vi "PCM Panel With Menu UI.vi"() -> ()   [LabVIEW 2016, in "PCM PanelSplit.lvclass"]
uses:
  PCM PanelSplit.lvclass
  PanelSplitToolkit/PanelObject/PanelObject.lvclass
  SubClass/PCM MenuVIPanelSplit.lvclass
  C:/Users/CL/Desktop/ZcDAQprj0811/ZcDAQprj/Modules/DAQ-Display/PanelSplitToolkit/PanelRootNode/PanelRootNode.lvclass
  PanelSplitToolkit/PanelDataNode/Split Mode.ctl
  <vilib>/Utility/error.llb/DialogType.ctl
  Display Mode.ctl
  <vilib>/Analysis/4window.llb/windowTd.ctl
  PanelSplitToolkit/PanelDataNode/PanelDataNode.lvclass
  <vilib>/Utility/miscctls.llb/LVRangeTypeDef.ctl
  PanelSplitToolkit/QueueManager.llb/CreatQueue.vi
  PanelSplitToolkit/QueueManager.llb/Insert.vi
  PanelSplitToolkit/QueueManager.llb/Remove.vi
  PanelSplitToolkit/QueueManager.llb/Destroy.vi
  PanelSplitToolkit/PanelRootNode/PanelRootNode.lvclass
  <vilib>/Analysis/NI_AALPro.lvlib
panel:
  in  "History":bool
  in  "Setting":bool
  in  "Float":bool
  in  "Close":bool
  in  "Node*":refnum<data-value>
  in  "down":bool
  in  "right":bool
  in  "left":bool
  in  "up":bool
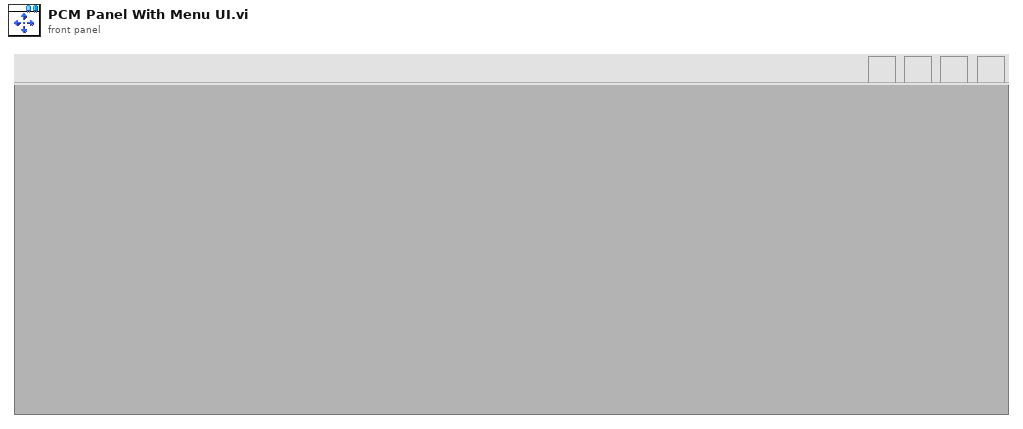
[diagram p1: front panel]
types:
  T1 = cluster{"Display[]":bool[], "error":errorcluster, "Float":bool}
  T2 = cluster{"error":errorcluster, "Event":string, "Data":variant, "Q_Local":string, "Caller":string, "SubPanel*":refnum<vi>, "RootNode*":refnum<data-value>, "Send":cluster{"SEvent":string, "SData":variant, "PanelNumber":i32}, "Arrow Button Refs":refnum<vi>[]}
  T3 = typedef "PanelDataNode.lvclass/Split Mode.ctl" = enum16{"Horizontal(up)", "Vertical(left)", "Horizontal(down)", "Vertical(right)"}
  T4 = typedef "LVPoint32TypeDef.ctl" = cluster{"Horizontal":i32, "Vertical":i32}
  T5 = typedef "PCM PanelSplit.lvclass/Display Mode.ctl" = enum16{"时域", "频谱", "功率谱"}
  T6 = enum32{"Invalid", "Standard", "Closed", "Hidden", "Minimized", "Maximized"}
  T7 = typedef "LVRangeTypeDef.ctl" = cluster{"Minimum":dbl, "Maximum":dbl, "Increment":dbl, "Minor Increment":dbl, "Start":dbl}
  T8 = typedef "DialogType.ctl" = u16
  T9 = typedef "PCM PanelSplit.lvclass/Display Config.ctl" = cluster{"Display Mode":T5, "ChTag[]":string[], "window":T10, "Range":T7}
  T10 = typedef "NI_AALPro.lvlib/windowTd.ctl" = u32
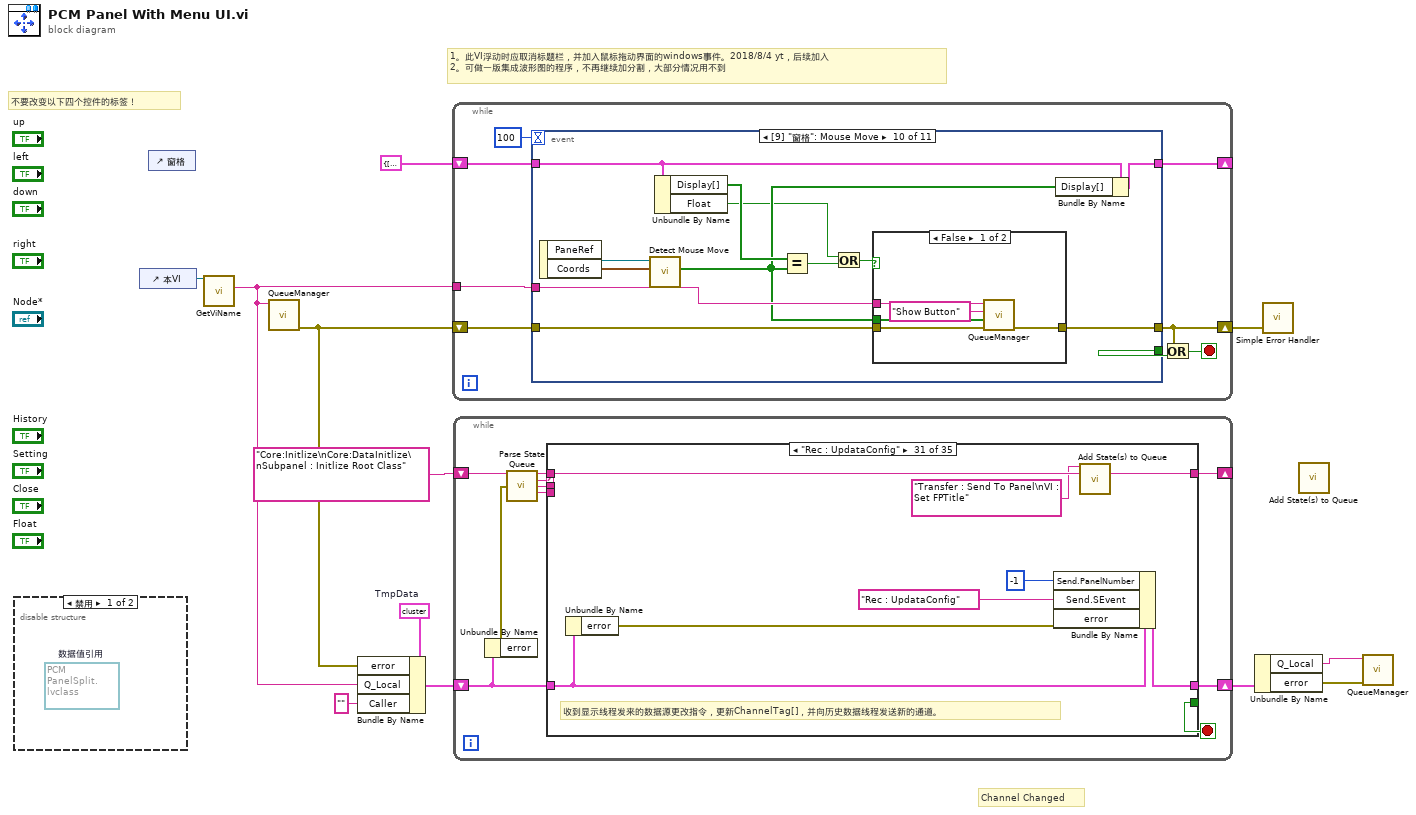
[diagram p0: block diagram]
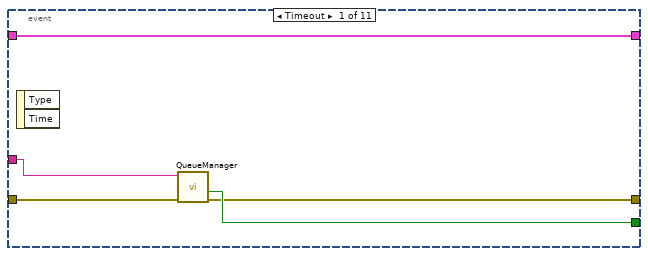
[diagram p3: hidden frame]
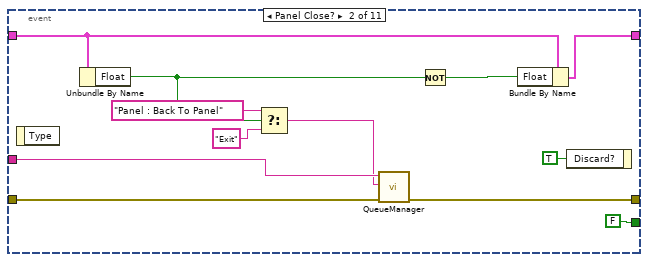
[diagram p4: hidden frame]
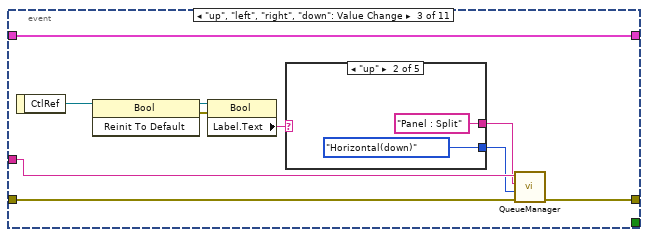
[diagram p5: hidden frame]
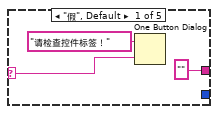
[diagram p6: hidden frame]
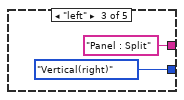
[diagram p7: hidden frame]
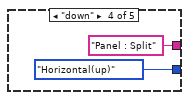
[diagram p8: hidden frame]
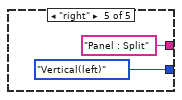
[diagram p9: hidden frame]
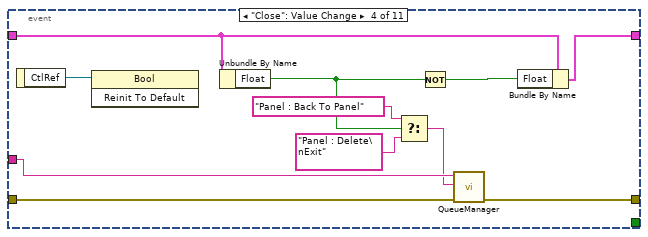
[diagram p10: hidden frame]
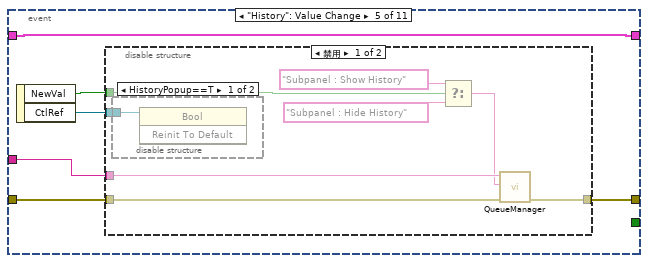
[diagram p11: hidden frame]
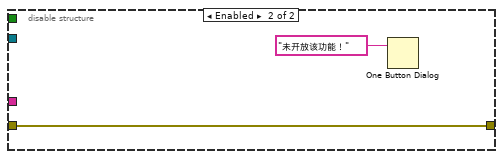
[diagram p13: hidden frame]
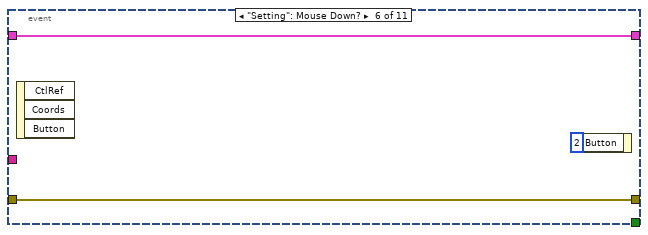
[diagram p14: hidden frame]
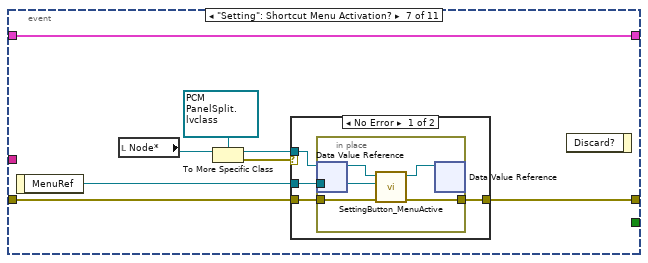
[diagram p15: hidden frame]
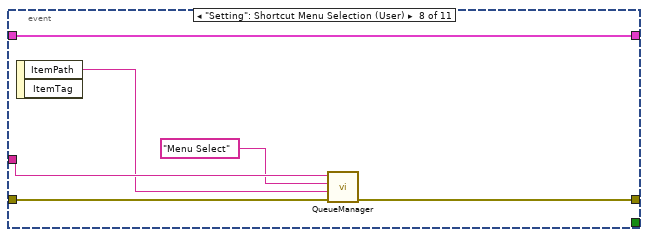
[diagram p17: hidden frame]
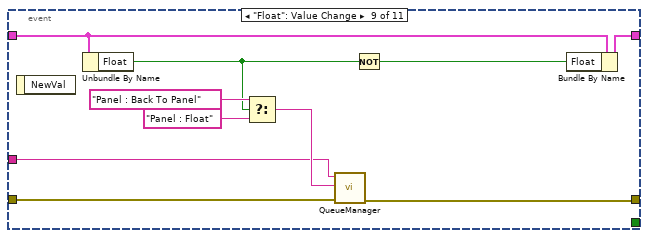
[diagram p18: hidden frame]
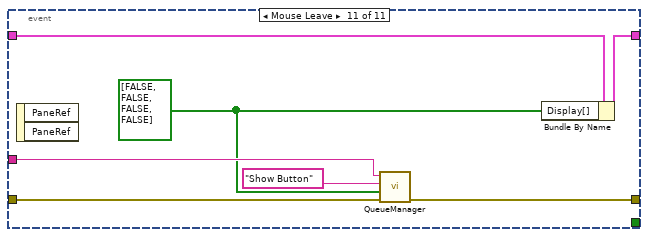
[diagram p20: hidden frame]
diagram:
  w8 = T2 {"error"={"status"=FALSE, "code"=0, "source"=""}, "Event"="", "Data"=variant, "Q_Local"="", "Caller"="", "SubPanel*"=refnum, "RootNode*"=refnum, "Send"={"SEvent"="", "SData"=variant, "PanelNumber"=-1}, "Arrow Button Refs"=[]}  # TmpData
  # "1。此VI浮动时应取消标题栏，并加入鼠标拖动界面的windows事件。2018/8/4 yt，后续加入\n2。可做一版集成波形图的程序，不再继续加分割，大部分情况用不到"
  # "Channel Changed"
  # "不要改变以下四个控件的标签！"
  n1 = disable-structure shown="禁用" {
    frame Disabled {
      (unwired) refnum<data-value> refnum  # 数据值引用
    }
    frame Enabled {
    }
  }
  n2 = control-ref of="本VI"() -> (w1:refnum<vi>)
  n3 = control-ref of="窗格"() -> ()  [unwired: 1 out]
  n4 = call "GetViName.vi"("VI*"=w1) -> ("VI Name"=w4:string)  [unwired: 9 in, 1 out]
  n5 = call-poly "QueueManager.vi"("QueueName"=w4) -> ("error out"=w3:errorcluster)  [unwired: 9 in, 1 out]
  n6 = Bundle By Name(cluster=w8, "error"=w3, "Q_Local"=w4, "Caller"="") -> (w7:T2)
  n7 = while {
    tunnel: w4 -> [w20]
    shift-right: [w16] -> w9
    shift-left: w3 -> [w19]
    shift-right: [w13] -> _
    shift-left: T1 {"Display[]"=[], "error"={"status"=FALSE, "code"=0, "source"=""}, "Float"=FALSE} -> [w14]
    stop <- w17 stop-if-true
    n8 = event shown="[9] \"窗格\": Mouse Move" {
      selector: _ -> [_ _ _ _ _ _ _ _ _ _ _]
      dyn-events: _ -> [_ _ _ _ _ _ _ _ _ _ _]
      timeout: 100 -> [_ _ _ _ _ _ _ _ _ _ _]
      tunnel: [w23 FALSE _ _ _ _ _ _ _ _ _] -> w18
      tunnel: w20 -> [w25 w36 w44 w67 w73 _ _ w111 w119 w133 w145]
      tunnel: w19 -> [w24 w35 w46 w69 w75 w88 w97 w113 w122 w132 w147]
      tunnel: [w22 w34 w45 w68 w74 w88 w96 w112 w121 w131 w146] -> w16
      tunnel: w14 -> [w21 w28 w38 w62 w71 w87 w90 w109 w118 w128 w144]
      tunnel: [w21 w27 w38 w61 w71 w87 w90 w109 w123 w127 w142] -> w13
      event Timeout {
        n9 = event-data() -> ()  [unwired: 1 in, 2 out]
        n10 = call-poly "QueueManager.vi"("error in (no error)"=w24, "Queue Name(unamed)"=w25) -> ("error out"=w22:errorcluster, "Not Exist?"=w23:bool)  [unwired: 8 in]
      }
      event Panel Close? {
        n11 = event-data() -> ()  [unwired: 1 in, 1 out]
        n12 = Unbundle By Name(w28) -> ("Float"=w26:bool)
        n13 = Select(t="Panel : Back To Panel", s=w26, f="Exit" ("Event")) -> (s? t:f=w30:string)
        n14 = call-poly "QueueManager.vi"("error in"=w35, "Event"=w30, "QueueName"=w36) -> ("error out"=w34:errorcluster)  [unwired: 7 in, 1 out]
        n15 = Not(x=w26) -> (.not. x?=w29:bool)
        n16 = Bundle By Name(cluster=w28, "Float"=w29) -> (w27:T1)
        n17 = event-data("Discard?"=TRUE ("放弃？")) -> ()  [unwired: 1 in, 1 out]
      }
      event "up", "left", "right", "down": Value Change {
        n18 = event-data() -> ("CtlRef"=w41:refnum<vi>)  [unwired: 1 in]
        n19 = invoke class="Bool" method="Reinit To Default"(reference=w41) -> (reference out=w43:refnum<vi>, error out=w42:errorcluster)  [unwired: 2 in, 1 out]
        n20 = property class="Bool"(reference=w43, error in=w42) -> ("Label.Text"=w47:string)  [unwired: 2 out]
        n21 = case shown="\"up\"" w47 {
          selector: w47 -> [w48 _ _ _ _]
          tunnel: [_ Split_Mode."Horizontal(down)" ("Split Mode") Split_Mode."Vertical(right)" ("Split Mode") Split_Mode."Horizontal(up)" ("Split Mode") Split_Mode."Vertical(left)" ("Split Mode")] -> w40
          tunnel: ["" "Panel : Split" "Panel : Split" "Panel : Split" "Panel : Split"] -> w39
          frame "假", Default {
            n22 = One Button Dialog(message="请检查控件标签！" ("消息"), button name ("OK")=w48) -> ()  [unwired: 1 out]
          }
          frame "up" {
          }
          frame "left" {
          }
          frame "down" {
          }
          frame "right" {
          }
        }
        n23 = call-poly "QueueManager.vi"("error in"=w46, "Data"=w40, "Event"=w39, "QueueName"=w44) -> ("error out"=w45:errorcluster)  [unwired: 6 in, 1 out]
      }
      event "Close": Value Change {
        n24 = event-data() -> ("CtlRef"=w66:refnum<vi>)  [unwired: 1 in]
        n25 = invoke class="Bool" method="Reinit To Default"(reference=w66) -> ()  [unwired: 2 in, 3 out]
        n26 = Unbundle By Name(w62) -> ("Float"=w60:bool)
        n27 = Select(t="Panel : Back To Panel" ("f"), s=w60, f="Panel : Delete\nExit" ("Event")) -> (s? t:f=w65:string)
        n28 = Not(x=w60) -> (.not. x?=w59:bool)
        n29 = call-poly "QueueManager.vi"("error in"=w69, "Event"=w65, "QueueName"=w67) -> ("error out"=w68:errorcluster)  [unwired: 7 in, 1 out]
        n30 = Bundle By Name(cluster=w62, "Float"=w59) -> (w61:T1)
      }
      event "History": Value Change {
        n31 = event-data() -> ("NewVal"=w72:bool, "CtlRef"=w70:refnum<vi>)  [unwired: 1 in]
        n32 = disable-structure shown="禁用" {
          disable-tunnel: w75 -> [w83 w86]
          disable-tunnel: [w82 w86] -> w74
          disable-tunnel: w73 -> [w81 _]
          disable-tunnel: w72 -> [w80 _]
          disable-tunnel: w70 -> [w76 _]
          frame Disabled {
            n33 = disable-structure shown="HistoryPopup==T" {
              disable-tunnel: w76 -> [w84 _]
              frame condition #0 {
                n34 = invoke class="Bool" method="Reinit To Default"(reference=w84) -> ()  [unwired: 2 in, 3 out]
              }
              frame condition #1 (active) {
              }
            }
            n35 = Select(t="Subpanel : Show History" ("Event"), s=w80, f="Subpanel : Hide History" ("Event")) -> (s? t:f=w77:string)
            n36 = call-poly "QueueManager.vi"("error in"=w83, "Event"=w77, "QueueName"=w81) -> ("error out"=w82:errorcluster)  [unwired: 7 in, 1 out]
          }
          frame Enabled {
            n37 = One Button Dialog(message="未开放该功能！" ("消息")) -> ()  [unwired: 1 in, 1 out]
          }
        }
      }
      event "Setting": Mouse Down? {
        n38 = event-data() -> ()  [unwired: 1 in, 3 out]
        n39 = event-data("Button"=u16 2 ("按钮")) -> ()  [unwired: 1 in, 1 out]
      }
      event "Setting": Shortcut Menu Activation? {
        n40 = event-data() -> ("MenuRef"=w95:refnum<k9>)  [unwired: 1 in]
        n41 = local read "Node*"() -> (w94:refnum<data-value>)
        n42 = To More Specific Class(target class=refnum<data-value> refnum ("数据值引用"), reference=w94) -> (specific class reference=w93:refnum<data-value>, error out=w91:errorcluster)  [unwired: 1 in]
        n43 = case shown="No Error" w91 {
          tunnel: w97 -> [w101 w107]
          tunnel: [w100 w107] -> w96
          tunnel: w95 -> [w99 _]
          tunnel: w93 -> [w98 _]
          frame No Error {
            n44 = in-place {
              in-place-border: w101 -> [w106]
              in-place-border: [w105] -> w100
              in-place-border: w99 -> [w104]
              n45 = in-place-dvr #1(w98) -> (w103:refnum<class "PCM PanelSplit.lvclass">)  [unwired: 1 out]
              n46 = call "SettingButton_MenuActive.vi"("error in"=w106, "Menu Ref"=w104, "PCM PanelSplit in"=w103) -> ("error out"=w105:errorcluster, "PCM PanelSplit out"=w102:refnum<class "PCM PanelSplit.lvclass">)  [unwired: 7 in]
              n47 = in-place-dvr #1(w102) -> ()  [unwired: 2 out]
            }
          }
          frame Error {
          }
        }
        n48 = event-data() -> ()  [unwired: 2 in, 1 out]
      }
      event "Setting": Shortcut Menu Selection (User) {
        n49 = event-data() -> ("ItemPath"=w108:string)  [unwired: 1 in, 1 out]
        n50 = call-poly "QueueManager.vi"("error in"=w113, "Data"=w108, "Event"="Menu Select", "QueueName"=w111) -> ("error out"=w112:errorcluster)  [unwired: 6 in, 1 out]
      }
      event "Float": Value Change {
        n51 = event-data() -> ()  [unwired: 1 in, 1 out]
        n52 = Unbundle By Name(w118) -> ("Float"=w115:bool)
        n53 = Select(t="Panel : Back To Panel", s=w115, f="Panel : Float" ("Event")) -> (s? t:f=w120:string)
        n54 = call-poly "QueueManager.vi"("error in"=w122, "Event"=w120, "QueueName"=w119) -> ("error out"=w121:errorcluster)  [unwired: 7 in, 1 out]
        n55 = Not(x=w115) -> (.not. x?=w114:bool)
        n56 = Bundle By Name(cluster=w118, "Float"=w114) -> (w123:T1)
      }
      event Mouse Move {
        n57 = event-data() -> ("PaneRef"=w135:refnum<vi>, "Coords"=w134:T4)  [unwired: 1 in]
        n58 = call "Detect Mouse Move.vi"("坐标"=w134, "窗格引用"=w135) -> ("Display[]"=w129:bool[])  [unwired: 9 in]
        n59 = Unbundle By Name(w128) -> ("Display[]"=w130:bool[], "Float"=w124:bool)
        n60 = Equal?(x=w130, y=w129) -> (x = y?=w125:bool)
        n61 = Or(x=w124, y=w125) -> (x .or. y?=w126:bool)
        n62 = case shown="False" w126 {
          tunnel: w133 -> [w140 _]
          tunnel: w132 -> [w139 w141]
          tunnel: [w138 w141] -> w131
          tunnel: w129 -> [w136 _]
          frame False {
            n63 = call-poly "QueueManager.vi"("error in"=w139, "Data"=w136, "Event"="Show Button", "QueueName"=w140) -> ("error out"=w138:errorcluster)  [unwired: 6 in, 1 out]
          }
          frame True {
          }
        }
        n64 = Bundle By Name(cluster=w128, "Display[]"=w129) -> (w127:T1)
      }
      event Mouse Leave {
        w143 = bool[] [FALSE, FALSE, FALSE, FALSE] ("Display[]")
        n65 = event-data() -> ()  [unwired: 1 in, 2 out]
        n66 = call-poly "QueueManager.vi"("error in"=w147, "Data"=w143, "Event"="Show Button", "QueueName"=w145) -> ("error out"=w146:errorcluster)  [unwired: 6 in, 1 out]
        n67 = Bundle By Name(cluster=w144, "Display[]"=w143) -> (w142:T1)
      }
    }
    n68 = Or(x=w16, y=w18) -> (x .or. y?=w17:bool)
  }
  n69 = while {
    shift-right: [w152] -> w10
    shift-left: w7 -> [w153]
    shift-right: [w151] -> _
    shift-left: "Core:Initlize\nCore:DataInitlize\nSubpanel : Initlize Root Class" -> [w158]
    stop <- w155 stop-if-true
    n70 = Unbundle By Name(w153) -> ("error"=w154:errorcluster)
    n71 = call "Parse State Queue.vi"("State Queue"=w158, "Error In (no error)"=w154) -> ("Remaining States"=w157:string, "Current State"=w156:string, "Arguments"=w150:string, "PreState"=w149:string)  [unwired: 10 in]
    n72 = case shown="\"Rec : UpdataConfig\"" w156 {
      selector: w156 -> [w160 _ _ _ _ _ _ _ _ _ _ _ _ _ _ _ _ _ _ _ _ _ _ _ _ _ _ _ _ _ _ _ _ _ _]
      tunnel: w157 -> [w165 w179 w198 w200 w209 w215 _ _ w244 w256 w267 w284 w293 w306 w320 w339 w345 w356 w360 w382 w400 w409 w426 w433 w446 w468 w478 w485 w487 w494 w516 w530 w538 w562 w571]
      tunnel: w150 -> [_ _ _ _ _ _ _ _ _ _ _ _ _ _ _ _ _ _ _ _ _ _ _ _ _ _ _ _ _ _ _ _ _ _ _]
      tunnel: [TRUE _ _ _ _ _ TRUE FALSE FALSE _ _ _ _ _ _ _ _ _ _ _ _ _ _ _ _ _ _ _ _ _ _ _ _ _ _] -> w155
      tunnel: w153 -> [w166 w176 w195 w199 w208 w217 w239 w242 w245 w248 w264 w280 w299 w308 w322 w329 w346 w350 w370 w375 w393 w410 w420 w432 w442 w464 w474 w486 w488 w496 w518 w521 w540 w556 w566]
      tunnel: [w166 w181 w194 w199 w206 w216 w239 w242 w245 w247 w263 w279 w297 w307 w321 w328 w346 w349 w369 w374 w392 w410 w419 w431 w441 w463 w473 w486 w488 w495 w517 w519 w539 w559 w565] -> w152
      tunnel: [w165 w178 w198 w200 w209 w214 "" ("Remaining States") "Subpanel : Destory\nCore:Exit" ("Remaining States") w244 w256 w267 w284 w292 w305 w319 w339 w345 w356 w359 w382 w400 w409 w426 w433 w446 w468 w478 w485 w487 w493 w515 w530 w538 w561 w571] -> w151
      tunnel: w149 -> [_ _ w192 _ _ _ _ _ _ _ _ _ _ _ _ _ _ _ _ _ _ _ _ _ _ _ _ _ _ _ _ _ _ _ _]
      frame "Default", Default {
        n73 = control-ref of="本VI"() -> (w161:refnum<vi>)
        n74 = call "GetViName.vi"("VI*"=w161) -> ("VI Name"=w159:string)  [unwired: 9 in, 1 out]
        n75 = Format Into String(format string="%s\n分支\"%s\"不存在！" ("格式字符串"), w159, w160) -> (resulting string=w164:string)  [unwired: 2 in, 1 out]
        n76 = One Button Dialog(message=w164) -> ()  [unwired: 1 in, 1 out]
      }
      frame "", "Idle" {
        n77 = Unbundle By Name(w176) -> ("Caller"=w170:string, "Q_Local"=w175:string, "error"=w174:errorcluster)
        n78 = Empty String/Path?(string/path=w170) -> (empty?=w173:bool)
        n79 = case shown="False" w173 {
          tunnel: [w184 FALSE ("Not Exist?")] -> w172
          tunnel: w170 -> [w183 _]
          frame False {
            n80 = call "Valid?.vi"("Queue Name(unamed)"=w183) -> ("Not Exist?"=w184:bool)  [unwired: 9 in, 1 out]
          }
          frame True {
          }
        }
        n81 = call-poly "QueueManager.vi"("Time out(-1)"=100, "error in (no error)"=w174, "Queue Name"=w175) -> ("error out"=w182:errorcluster, "Data"=w180:variant, "Event"=w169:string)  [unwired: 5 in, 1 out]
        n82 = Select(t="Exit" ("Event"), s=w172, f="") -> (s? t:f=w167:string)
        n83 = call "Add State(s) to Queue.vi"("State(s) in Front (\"\")"=w167, "State(s) in (\"\")"=w179, "State(s) at Back (\"\")"=w169) -> ("States Out"=w178:string)  [unwired: 12 in]
        n84 = Bundle By Name(cluster=w176, "Data"=w180, "error"=w182) -> (w181:T2)
      }
      frame "Error Handler" {
        w193 = T8 2 items=["无对话框", "确定信息", "继续或停止信息", "确定信息＋警告", "继续/停止+警告"] ("type of dialog (OK msg:1)")
        # "不要更改本分支名称！"
        n85 = Unbundle By Name(w195) -> ("error"=w187:errorcluster)
        n86 = Unbundle By Name(w187) -> ("source"=w190:string)
        n87 = Concatenate Strings("产生错误的分支：" ("字符串"), w192, "\n", w190) -> (w188:string)
        n88 = Bundle By Name(cluster=w187, "source"=w188) -> (w186:errorcluster)
        n89 = call <vilib>:"Simple Error Handler.vi"("type of dialog (OK msg:1)"=w193, "error in (no error)"=w186) -> ("error out"=w196:errorcluster)  [unwired: 3 in, 4 out]
        n90 = call <vilib>:"Clear Errors.vi"("error in (no error)"=w196) -> ("error out"=w197:errorcluster)  [unwired: 5 in, 1 out]
        n91 = Bundle By Name(cluster=w195, "error"=w197) -> (w194:T2)
      }
      frame "Core:Initlize" {
      }
      frame "Core:DataInitlize" {
        n92 = control-ref of="left"() -> (w202:refnum<vi>)
        n93 = control-ref of="down"() -> (w203:refnum<vi>)
        n94 = control-ref of="right"() -> (w201:refnum<vi>)
        n95 = control-ref of="up"() -> (w204:refnum<vi>)
        n96 = Build Array(w204, w203, w202, w201) -> (w205:refnum<vi>[])
        n97 = for {
          tunnel: w205 -> [w211] mode=indexing
          n98 = property class="Bool"(reference=w211, "Visible"=FALSE ("可见")) -> ()  [unwired: 1 in, 2 out]
        }
        n99 = control-ref of="子面板"() -> (w207:refnum<vi>)
        n100 = Bundle By Name(cluster=w208, "Arrow Button Refs"=w205, "SubPanel*"=w207) -> (w206:T2)
      }
      frame "Load" {
        n101 = local read "Node*"() -> (w219:refnum<data-value>)
        n102 = Unbundle By Name(w217) -> ("error"=w218:errorcluster)
        n103 = To More Specific Class(target class=refnum<data-value> refnum ("数据值引用"), reference=w219, error in=w218) -> (specific class reference=w220:refnum<data-value>, error out=w212:errorcluster)
        n104 = case shown="No Error" w212 {
          tunnel: w212 -> [w230 _]
          tunnel: w220 -> [w229 _]
          tunnel: w217 -> [w228 w237]
          tunnel: [w227 w237] -> w216
          tunnel: ["Transfer : Send To Panel\nVI : Set FPTitle" ("State(s) in Front (\"\")") "" ("State(s) in Front (\"\")")] -> w213
          frame No Error {
            n105 = in-place {
              in-place-border: w230 -> [w231]
              in-place-border: [w233] -> w226
              in-place-border: [w232] -> w225
              n106 = in-place-dvr #2(w229) -> (w235:refnum<class "PCM PanelSplit.lvclass">)  [unwired: 1 out]
              n107 = call "Read DisplayConfig.vi"("error in"=w231, "PCM PanelSplit 输入"=w235) -> ("error out"=w233:errorcluster, "Display Config"=w232:T9, "PCM PanelSplit 输出"=w234:refnum<class "PCM PanelSplit.lvclass">)  [unwired: 7 in]
              n108 = in-place-dvr #2(w234) -> ()  [unwired: 2 out]
            }
            n109 = Bundle By Name(cluster=w228, "Send.PanelNumber"=-1, "Send.SEvent"="Rec : Load", "Send.SData"=w225, "error"=w226) -> (w227:T2)
          }
          frame Error {
          }
        }
        n110 = call "Add State(s) to Queue.vi"("State(s) in Front (\"\")"=w213, "State(s) in (\"\")"=w215) -> ("States Out"=w214:string)  [unwired: 13 in]
      }
      frame "Core:Exit" {
      }
      frame "Exit" {
      }
      frame "-----User Event------" {
      }
      frame "Show Button" {
        n111 = Unbundle By Name(w248) -> ("Arrow Button Refs"=w252:refnum<vi>[], "Data"=w254:variant, "error"=w255:errorcluster)
        n112 = Variant To Data(error in=w255, type=bool[] [] ("Display[]"), Variant=w254) -> (data=w251:bool[], error out=w250:errorcluster)
        n113 = for {
          tunnel: w252 -> [w260] mode=indexing
          tunnel: w251 -> [w259] mode=indexing
          tunnel: w250 -> [w258]
          tunnel: [w257] -> w249
          n114 = property class="Bool"(reference=w260, error in=w258, "Visible"=w259) -> (error out=w257:errorcluster)  [unwired: 1 out]
        }
        n115 = Bundle By Name(cluster=w248, "error"=w249) -> (w247:T2)
      }
      frame "Hide Buttons" {
        n116 = Unbundle By Name(w264) -> ("Arrow Button Refs"=w266:refnum<vi>[], "error"=w262:errorcluster)  [unwired: 1 out]
        n117 = for {
          tunnel: w266 -> [w271] mode=indexing
          tunnel: FALSE -> [w270]
          tunnel: w262 -> [w269]
          tunnel: [w268] -> w265
          n118 = property class="Bool"(reference=w271, error in=w269, "Visible"=w270) -> (error out=w268:errorcluster)  [unwired: 1 out]
        }
        n119 = Bundle By Name(cluster=w264, "error"=w265) -> (w263:T2)
      }
      frame "Menu Select" {
        n120 = Unbundle By Name(w280) -> ("Q_Local"=w272:string, "Data"=w283:variant, "error"=w282:errorcluster)
        n121 = Variant To Data(error in=w282, type=w272, Variant=w283) -> (data=w273:string, error out=w281:errorcluster)
        n122 = local read "Node*"() -> (w278:refnum<data-value>)
        n123 = To More Specific Class(target class=refnum<data-value> refnum ("数据值引用"), reference=w278, error in=w281) -> (specific class reference=w277:refnum<data-value>, error out=w276:errorcluster)
        n124 = in-place {
          in-place-border: w276 -> [w290]
          in-place-border: [w288] -> w274
          in-place-border: w273 -> [w286]
          in-place-border: w272 -> [w285]
          n125 = in-place-dvr #3(w277) -> (w289:refnum<class "PCM PanelSplit.lvclass">)  [unwired: 1 out]
          n126 = call "SettingButton_MenuSelect by Path.vi"("error in (no error)"=w290, "QName"=w285, "MenuPath"=w286, "PCM PanelSplit 输入"=w289) -> ("error out"=w288:errorcluster, "PCM PanelSplit 输出"=w287:refnum<class "PCM PanelSplit.lvclass">)  [unwired: 6 in]
          n127 = in-place-dvr #3(w287) -> ()  [unwired: 2 out]
        }
        n128 = Bundle By Name(cluster=w280, "error"=w274) -> (w279:T2)
      }
      frame "DisplayMode Changed" {
        n129 = Unbundle By Name(w299) -> ("Data"=w301:variant, "error"=w302:errorcluster)
        n130 = Variant To Data(error in=w302, type=Display_Mode."时域" ("Display Mode"), Variant=w301) -> (data=w294:T5, error out=w298:errorcluster)
        n131 = Bundle By Name(cluster=w299, "Send.PanelNumber"=-1, "Send.SEvent"="Rec : DisplayMode Changed", "Send.SData"=w294, "error"=w298) -> (w297:T2)
        n132 = call "Add State(s) to Queue.vi"("State(s) in Front (\"\")"="Transfer : Send To Panel\nVI : Set FPTitle" ("State(s) in Front (\"\")"), "State(s) in (\"\")"=w293) -> ("States Out"=w292:string)  [unwired: 13 in]
      }
      frame "Channel Changed" {
        n133 = Unbundle By Name(w308) -> ("Event"=w313:string, "Data"=w314:variant, "error"=w315:errorcluster)
        n134 = Build Array(w313) -> (w312:string[])
        n135 = Variant To Data(error in=w315, type=w312, Variant=w314) -> (data=w303:string[], error out=w309:errorcluster)
        n136 = Bundle By Name(cluster=w308, "Send.PanelNumber"=-1, "Send.SEvent"="Rec : Channel Changed", "Send.SData"=w303, "error"=w309) -> (w307:T2)
        n137 = call "Add State(s) to Queue.vi"("State(s) in Front (\"\")"="Transfer : Send To Panel\nVI : Set FPTitle" ("State(s) in Front (\"\")"), "State(s) in (\"\")"=w306) -> ("States Out"=w305:string)  [unwired: 13 in]
      }
      frame "Window Changed" {
        w316 = T10 1 items=["矩形"=0, "Hanning"=1, "Hamming"=2, "Blackman-Harris"=3, "Exact Blackman"=4, "Blackman"=5, "Flat Top"=6, "4阶Blackman-Harris "=7, "7阶Blackman-Harris"=8, "Low Sidelobe"=9, "Blackman Nuttall"=11, "三角"=30, "Bartlett-Hanning"=31, "Bohman"=32, "Parzen"=33, "Welch"=34, "Kaiser"=60, "Dolph-Chebyshev"=61, "高斯"=62] ("window")
        n138 = Unbundle By Name(w322) -> ("Data"=w326:variant, "error"=w327:errorcluster)
        n139 = Variant To Data(error in=w327, type=w316, Variant=w326) -> (data=w317:T10, error out=w323:errorcluster)
        n140 = Bundle By Name(cluster=w322, "Send.PanelNumber"=-1, "Send.SEvent"="Rec : Window Changed", "Send.SData"=w317, "error"=w323) -> (w321:T2)
        n141 = call "Add State(s) to Queue.vi"("State(s) in Front (\"\")"="Transfer : Send To Panel\nVI : Set FPTitle" ("State(s) in Front (\"\")"), "State(s) in (\"\")"=w320) -> ("States Out"=w319:string)  [unwired: 13 in]
      }
      frame "VI : Set FPTitle" {
        n142 = Unbundle By Name(w329) -> ("error"=w331:errorcluster)
        n143 = local read "Node*"() -> (w338:refnum<data-value>)
        n144 = To More Specific Class(target class=refnum<data-value> refnum ("数据值引用"), reference=w338, error in=w331) -> (specific class reference=w337:refnum<data-value>, error out=w335:errorcluster)
        n145 = in-place {
          in-place-border: w335 -> [_]
          in-place-border: [w341] -> w334
          in-place-border: [w340] -> w333
          n146 = in-place-dvr #4(w337) -> (w344:refnum<class "PCM PanelSplit.lvclass">, w343:errorcluster)
          n147 = call "Get Information String.vi"("error in (no error)"=w343, "PCM PanelSplit.lvclass"=w344) -> ("error out"=w340:errorcluster, "Information String out"=w341:string, "PCM PanelSplit out"=w342:refnum<class "PCM PanelSplit.lvclass">)  [unwired: 7 in]
          n148 = in-place-dvr #4(w342) -> ()  [unwired: 2 out]
        }
        n149 = control-ref of="本VI"() -> (w332:refnum<vi>)
        n150 = property class="VI"(reference=w332, error in=w333, "Front Panel.Title"=w334) -> (error out=w330:errorcluster)  [unwired: 1 out]
        n151 = Bundle By Name(cluster=w329, "error"=w330) -> (w328:T2)
      }
      frame "----Main Panel Action-------" {
      }
      frame "Panel : Delete" {
        n152 = Unbundle By Name(w350) -> ("error"=w348:errorcluster)
        n153 = local read "Node*"() -> (w354:refnum<data-value>)
        n154 = To More Specific Class(target class=refnum<data-value> refnum ("Node*"), reference=w354, error in=w348) -> (specific class reference=w353:refnum<data-value>, error out=w347:errorcluster)
        n155 = call "Q_Delete.vi"("error in"=w347, "CloseVI?(T)"=FALSE, "ChildNode*"=w353) -> ("error out"=w351:errorcluster)  [unwired: 8 in]
        n156 = Bundle By Name(cluster=w350, "error"=w351) -> (w349:T2)
      }
      frame "Panel : Split" {
        n157 = Unbundle By Name(w370) -> ("Data"=w366:variant, "error"=w365:errorcluster)
        n158 = Variant To Data(error in=w365, type=Split_Mode."Horizontal(up)" ("Split Mode"), Variant=w366) -> (data=w363:T3, error out=w362:errorcluster)
        n159 = local read "Node*"() -> (w371:refnum<data-value>)
        n160 = To More Specific Class(target class=refnum<data-value> refnum ("Node*"), reference=w371, error in=w362) -> (specific class reference=w367:refnum<data-value>, error out=w361:errorcluster)
        n161 = call "Q_Split.vi"("error in"=w361, "Split Mode"=w363, "ChildNode*"=w367) -> ("error out"=w368:errorcluster)  [unwired: 8 in]
        n162 = Wait (ms)(milliseconds to wait=u32 50 ("等待时间（毫秒）")) -> ()  [unwired: 1 out]
        n163 = call "Add State(s) to Queue.vi"("State(s) in (\"\")"=w360, "State(s) at Back (\"\")"="Hide Buttons" ("State(s) at Back (\"\")")) -> ("States Out"=w359:string)  [unwired: 13 in]
        n164 = Bundle By Name(cluster=w370, "error"=w368) -> (w369:T2)
      }
      frame "Panel : Back To Panel" {
        n165 = Unbundle By Name(w375) -> ("error"=w377:errorcluster)
        n166 = local read "Node*"() -> (w381:refnum<data-value>)
        n167 = To More Specific Class(target class=refnum<data-value> refnum ("Node*"), reference=w381) -> (specific class reference=w379:refnum<data-value>, error out=w378:errorcluster)  [unwired: 1 in]
        n168 = case shown="No Error" w378 {
          tunnel: w377 -> [w385 w390]
          tunnel: [w384 w390] -> w376
          tunnel: w379 -> [w383 _]
          frame No Error {
            n169 = in-place {
              in-place-border: w385 -> [w387]
              in-place-border: [w386] -> w384
              n170 = in-place-dvr #5(w383) -> (w389:refnum<class "PanelDataNode.lvclass">)  [unwired: 1 out]
              n171 = call "BackToPanel.vi"("error in (no error)"=w387, "PanelDataNode 输入"=w389) -> ("error out"=w386:errorcluster, "PanelDataNode 输出"=w388:refnum<class "PanelDataNode.lvclass">)  [unwired: 8 in]
              n172 = in-place-dvr #5(w388) -> ()  [unwired: 2 out]
            }
          }
          frame Error {
          }
        }
        n173 = local write "Float"(FALSE ("Float")) -> ()
        n174 = Bundle By Name(cluster=w375, "error"=w376) -> (w374:T2)
      }
      frame "Panel : Float" {
        n175 = Unbundle By Name(w393) -> ("error"=w395:errorcluster)
        n176 = local read "Node*"() -> (w399:refnum<data-value>)
        n177 = To More Specific Class(target class=refnum<data-value> refnum ("Node*"), reference=w399) -> (specific class reference=w397:refnum<data-value>, error out=w396:errorcluster)  [unwired: 1 in]
        n178 = case shown="No Error" w396 {
          tunnel: w395 -> [w403 w408]
          tunnel: [w402 w408] -> w394
          tunnel: w397 -> [w401 _]
          frame No Error {
            n179 = in-place {
              in-place-border: w403 -> [w407]
              in-place-border: [w406] -> w402
              n180 = in-place-dvr #6(w401) -> (w405:refnum<class "PanelDataNode.lvclass">)  [unwired: 1 out]
              n181 = call "FloatPanel.vi"("error in (no error)"=w407, "PanelDataNode 输入"=w405) -> ("error out"=w406:errorcluster, "PanelDataNode 输出"=w404:refnum<class "PanelDataNode.lvclass">)  [unwired: 8 in]
              n182 = in-place-dvr #6(w404) -> ()  [unwired: 2 out]
            }
          }
          frame Error {
          }
        }
        n183 = local write "Float"(TRUE ("Float")) -> ()
        n184 = Bundle By Name(cluster=w393, "error"=w394) -> (w392:T2)
      }
      frame "----Local Subpanel Action----" {
      }
      frame "Subpanel : Initlize Root Class" {
        n185 = Unbundle By Name(w420) -> ("SubPanel*"=w417:refnum<vi>, "Q_Local"=w422:string, "error"=w418:errorcluster)
        n186 = control-ref of="本VI"() -> (w421:refnum<vi>)
        n187 = To More Specific Class(target class=refnum<vi> refnum ("RootPanel"), reference=w417, error in=w418) -> (specific class reference=w424:refnum<vi>, error out=w423:errorcluster)
        n188 = call-dynamic "Initialize Root.vi"("RootQueueName"=w422, "error in (no error)"=w423, "CurrentVi*"=w421, "RootPanel*"=w424, "PCM MenuVIPanelSplit 输入"=refnum<class "PCM MenuVIPanelSplit.lvclass"> refnum ("PCM MenuVIPanelSplit.lvclass")) -> ("error out"=w412:errorcluster, "SelfNode*"=w415:refnum<data-value>)  [unwired: 5 in]
        n189 = To More Specific Class(target class=refnum<data-value> refnum ("RootNode*"), reference=w415, error in=w412) -> (specific class reference=w413:refnum<data-value>, error out=w411:errorcluster)
        n190 = Bundle By Name(cluster=w420, "RootNode*"=w413, "error"=w411) -> (w419:T2)
      }
      frame "Subpanel : Change Graph" {
        # "切换用于实时显示VI（时域、频谱、功率谱等）"
        n191 = Unbundle By Name(w432) -> ("RootNode*"=w429:refnum<data-value>, "Data"=w427:variant, "error"=w428:errorcluster)  [unwired: 1 out]
        n192 = in-place {
          in-place-border: w428 -> [w438]
          in-place-border: [w437] -> w430
          in-place-border: w427 -> [w435]
          n193 = in-place-dvr #7(w429) -> (w439:refnum<class "PCM MenuVIPanelSplit.lvclass">)  [unwired: 1 out]
          n194 = call-dynamic "Change Insert VI.vi"("Abort Original VI"=TRUE ("Abort Originally VI"), "error in"=w438, "Data"=w435, "PanelRootNode in"=w439) -> ("error out"=w437:errorcluster, "PanelRootNode out"=w436:refnum<class "PCM MenuVIPanelSplit.lvclass">)  [unwired: 6 in]
          n195 = in-place-dvr #7(w436) -> ()  [unwired: 2 out]
        }
        n196 = Bundle By Name(cluster=w432, "error"=w430) -> (w431:T2)
      }
      frame "Subpanel : Show History" {
        # "显示或隐藏历史曲线"
        n197 = Unbundle By Name(w442) -> ("RootNode*"=w444:refnum<data-value>, "Q_Local"=w440:string, "error"=w443:errorcluster)
        n198 = disable-structure shown="默认" {
          disable-tunnel: [w450 w456] -> w445
          disable-tunnel: w444 -> [w449 w461]
          disable-tunnel: w443 -> [w448 w455]
          disable-tunnel: w440 -> [w447 _]
          frame condition #0 (active) {
            n199 = in-place {
              in-place-border: w448 -> [w454]
              in-place-border: [w453] -> w450
              in-place-border: w447 -> [_]
              n200 = in-place-dvr #8(w449) -> (w452:refnum<class "PCM MenuVIPanelSplit.lvclass">)  [unwired: 1 out]
              n201 = call "ShowHistoryGraph.vi"("error in"=w454, "PCM MenuVIPanelSplit.lvclass"=w452) -> ("error out"=w453:errorcluster, "PCM MenuVIPanelSplit.lvclass out"=w451:refnum<class "PCM MenuVIPanelSplit.lvclass">)  [unwired: 8 in]
              n202 = in-place-dvr #8(w451) -> ()  [unwired: 2 out]
            }
          }
          frame condition #1 {
            n203 = vi-ref "HistoryGraph.vi"() -> (w462:refnum<vi>)
            n204 = call "Dynamic Load by Ref.vi"("error in"=w455, "CtrlValue"=w461, "CtrlName"="Node*", "Static vi reference in"=w462) -> ("错误输出"=w457:errorcluster, "Dynamic vi reference out"=w459:refnum<vi>)  [unwired: 6 in]
            n205 = invoke class="VI" method="FP.Open"(reference=w459, error in=w457, "State"=T6."Standard" ("状态")) -> (error out=w456:errorcluster)  [unwired: 2 in, 4 out]
          }
        }
        n206 = Bundle By Name(cluster=w442, "error"=w445) -> (w441:T2)
      }
      frame "Subpanel : Hide History" {
        # "显示或隐藏历史曲线"
        n207 = Unbundle By Name(w464) -> ("RootNode*"=w466:refnum<data-value>, "error"=w465:errorcluster)  [unwired: 2 out]
        n208 = in-place {
          in-place-border: w465 -> [w472]
          in-place-border: [w471] -> w467
          n209 = in-place-dvr #9(w466) -> (w470:refnum<class "PCM MenuVIPanelSplit.lvclass">)  [unwired: 1 out]
          n210 = call "HideHistoryGraph.vi"("error in"=w472, "PCM MenuVIPanelSplit.lvclass"=w470) -> ("error out"=w471:errorcluster, "PCM MenuVIPanelSplit.lvclass out"=w469:refnum<class "PCM MenuVIPanelSplit.lvclass">)  [unwired: 8 in]
          n211 = in-place-dvr #9(w469) -> ()  [unwired: 2 out]
        }
        n212 = Bundle By Name(cluster=w464, "error"=w467) -> (w463:T2)
      }
      frame "Subpanel : Destory" {
        n213 = Unbundle By Name(w474) -> ("RootNode*"=w476:refnum<data-value>, "error"=w475:errorcluster)
        n214 = in-place {
          in-place-border: w475 -> [w480]
          in-place-border: [w484] -> w477
          n215 = in-place-dvr #10(w476) -> (w483:refnum<class "PCM MenuVIPanelSplit.lvclass">, w481:errorcluster)
          n216 = Merge Errors(w481, w480) -> (w479:errorcluster)
          n217 = call-dynamic "Destory.vi"("error in (no error)"=w479, "PanelRootNode 输入"=w483) -> ("error out"=w484:errorcluster, "PanelRootNode 输出"=w482:refnum<class "PCM MenuVIPanelSplit.lvclass">)  [unwired: 8 in]
          n218 = in-place-dvr #10(w482) -> ()  [unwired: 2 out]
        }
        n219 = Bundle By Name(cluster=w474, "error"=w477) -> (w473:T2)
      }
      frame "----Communication----" {
      }
      frame "Rec : Request Channel Info" {
      }
      frame "Rec : Source Changed" {
        # "收到显示线程发来的数据源更改指令，更新ChannelTag[]，并向历史数据线程发送新的通道。"
        n220 = Unbundle By Name(w496) -> ("Data"=w490:variant, "error"=w505:errorcluster)
        n221 = local read "Node*"() -> (w501:refnum<data-value>)
        n222 = Variant To Data(error in=w505, type=string[] [], Variant=w490) -> (data=w499:string[], error out=w500:errorcluster)
        n223 = To More Specific Class(target class=refnum<data-value> refnum ("数据值引用"), reference=w501, error in=w500) -> (specific class reference=w504:refnum<data-value>, error out=w503:errorcluster)
        n224 = in-place {
          in-place-border: w503 -> [w508]
          in-place-border: w499 -> [w507]
          in-place-border: [w506] -> w497
          n225 = in-place-dvr #11(w504) -> (w510:refnum<class "PCM PanelSplit.lvclass">)  [unwired: 1 out]
          n226 = call-dynamic "PCM Attribute Set DisplayTags.vi"("error in (no error)"=w508, "Display CH Tag[]"=w507, "PCM PanelSplit 输入"=w510) -> ("error out"=w506:errorcluster, "PCM PanelSplit 输出"=w509:refnum<class "PCM PanelSplit.lvclass">)  [unwired: 7 in]
          n227 = in-place-dvr #11(w509) -> ()  [unwired: 2 out]
        }
        n228 = Bundle By Name(cluster=w496, "Send.PanelNumber"=1, "Send.SEvent"="Rec : Channel Changed", "Send.SData"=w490, "error"=w497) -> (w495:T2)
        n229 = call "Add State(s) to Queue.vi"("State(s) in Front (\"\")"="Transfer : Send To Panel\nVI : Set FPTitle" ("State(s) in Front (\"\")"), "State(s) in (\"\")"=w494) -> ("States Out"=w493:string)  [unwired: 13 in]
      }
      frame "Rec : UpdataConfig" {
        # "收到显示线程发来的数据源更改指令，更新ChannelTag[]，并向历史数据线程发送新的通道。"
        n230 = Unbundle By Name(w518) -> ("error"=w511:errorcluster)
        n231 = Bundle By Name(cluster=w518, "Send.PanelNumber"=-1, "Send.SEvent"="Rec : UpdataConfig", "error"=w511) -> (w517:T2)
        n232 = call "Add State(s) to Queue.vi"("State(s) in Front (\"\")"="Transfer : Send To Panel\nVI : Set FPTitle" ("State(s) in Front (\"\")"), "State(s) in (\"\")"=w516) -> ("States Out"=w515:string)  [unwired: 13 in]
      }
      frame "Rec : YScaleChanged" {
        n233 = Unbundle By Name(w521) -> ("Data"=w528:variant, "error"=w529:errorcluster)
        n234 = Variant To Data(error in=w529, type=T7 {"Minimum"=0.0, "Maximum"=0.0, "Increment"=0.0, "Minor Increment"=0.0, "Start"=0.0} ("Y标尺.范围"), Variant=w528) -> (data=w522:T7, error out=w523:errorcluster)
        n235 = local read "Node*"() -> (w524:refnum<data-value>)
        n236 = To More Specific Class(target class=refnum<data-value> refnum ("数据值引用"), reference=w524) -> (specific class reference=w525:refnum<data-value>)  [unwired: 1 in, 1 out]
        n237 = in-place {
          in-place-border: w523 -> [w535]
          in-place-border: [w534] -> w520
          in-place-border: w522 -> [w531]
          n238 = in-place-dvr #12(w525) -> (w533:refnum<class "PCM PanelSplit.lvclass">)  [unwired: 1 out]
          n239 = call-dynamic "PCM Attribute Set YScale.vi"("error in (no error)"=w535, "Range"=w531, "PCM PanelSplit 输入"=w533) -> ("error out"=w534:errorcluster, "PCM PanelSplit 输出"=w532:refnum<class "PCM PanelSplit.lvclass">)  [unwired: 7 in]
          n240 = in-place-dvr #12(w532) -> ()  [unwired: 2 out]
        }
        n241 = Bundle By Name(cluster=w521, "error"=w520) -> (w519:T2)
      }
      frame "Response : CH Tags" {
        # "向请求通道列表的线程发送当前通道"
        n242 = Unbundle By Name(w540) -> ("Event"=w541:string, "Data"=w546:variant, "error"=w545:errorcluster)
        n243 = local read "Node*"() -> (w549:refnum<data-value>)
        n244 = Variant To Data(error in=w545, type=w541, Variant=w546) -> (data=w542:string, error out=w544:errorcluster)
        n245 = To More Specific Class(target class=refnum<data-value> refnum ("数据值引用"), reference=w549) -> (specific class reference=w547:refnum<data-value>)  [unwired: 1 in, 1 out]
        n246 = in-place {
          in-place-border: [w550] -> w543
          n247 = in-place-dvr #13(w547) -> (w554:refnum<class "PCM PanelSplit.lvclass">, w553:errorcluster)
          n248 = call "Read DisplayConfig.vi"("error in"=w553, "PCM PanelSplit 输入"=w554) -> ("Display Config"=w551:T9, "PCM PanelSplit 输出"=w552:refnum<class "PCM PanelSplit.lvclass">)  [unwired: 7 in, 1 out]
          n249 = Unbundle By Name(w551) -> ("ChTag[]"=w550:string[])
          n250 = in-place-dvr #13(w552) -> ()  [unwired: 2 out]
        }
        n251 = call-poly "QueueManager.vi"("error in"=w544, "Data"=w543, "QueueName"=w542) -> ("error out"=w537:errorcluster)  [unwired: 7 in, 1 out]
        n252 = call <vilib>:"Clear Errors.vi"("error in (no error)"=w537) -> ("error out"=w536:errorcluster)  [unwired: 5 in, 1 out]
        n253 = Bundle By Name(cluster=w540, "error"=w536) -> (w539:T2)
      }
      frame "Transfer : Send QName" {
        n254 = Unbundle By Name(w556) -> ("Q_Local"=w555:string)
        n255 = Bundle By Name(cluster=w556, "Send.PanelNumber"=-1, "Send.SEvent"="", "Send.SData"=w555) -> (w559:T2)
        n256 = call "Add State(s) to Queue.vi"("State(s) in Front (\"\")"="Transfer : Send To Panel", "State(s) in (\"\")"=w562) -> ("States Out"=w561:string)  [unwired: 13 in]
      }
      frame "Transfer : Send To Panel" {
        n257 = Unbundle By Name(w566) -> ("RootNode*"=w569:refnum<data-value>, "Send.PanelNumber"=w563:i32, "Send.SEvent"=w564:string, "Send.SData"=w567:variant, "error"=w568:errorcluster)
        n258 = in-place {
          in-place-border: w568 -> [w578]
          in-place-border: [w577] -> w570
          in-place-border: w567 -> [w573]
          in-place-border: w564 -> [w574]
          in-place-border: w563 -> [w572]
          n259 = in-place-dvr #14(w569) -> (w576:refnum<class "PCM MenuVIPanelSplit.lvclass">)  [unwired: 1 out]
          n260 = call "SendToPanels.vi"("PanelNumber(-1)"=w572, "error in"=w578, "Data"=w573, "Event"=w574, "PanelRootNode in"=w576) -> ("error out"=w577:errorcluster, "PanelRootNode out"=w575:refnum<class "PCM MenuVIPanelSplit.lvclass">)  [unwired: 5 in]
          n261 = in-place-dvr #14(w575) -> ()  [unwired: 2 out]
        }
        n262 = Bundle By Name(cluster=w566, "error"=w570) -> (w565:T2)
      }
    }
  }
  n263 = Unbundle By Name(w10) -> ("Q_Local"=w6:string, "error"=w11:errorcluster)
  n264 = call <vilib>:"Simple Error Handler.vi"("error in (no error)"=w9) -> ()  [unwired: 4 in, 5 out]
  n265 = call "Add State(s) to Queue.vi"() -> ()  [unwired: 15 in, 1 out]
  n266 = call-poly "QueueManager.vi"("error in (no error)"=w11, "QueeuName"=w6) -> ()  [unwired: 9 in, 1 out]
